vi "Test Upload to S3.vi"() -> ()   [LabVIEW 2019, in "SMO.Control Experiment.lvclass"]
uses:
  SMO.Control Experiment.lvclass
panel:
  out "Control Experiment out":refnum<class "SMO.Control Experiment.lvclass">
  in  "Control Experiment":refnum<class "SMO.Control Experiment.lvclass">
  in  "file to upload":path
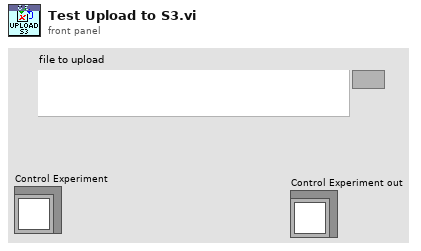
[diagram p1: front panel]
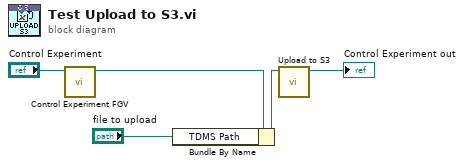
[diagram p0: block diagram]
diagram:
  n1 = call "Control Experiment FGV.vi"("Control Experiment"="Control Experiment") -> ("Control Experiment out"=w3:refnum<class "SMO.Control Experiment.lvclass">)  [unwired: 9 in, 1 out]
  n2 = Bundle By Name(cluster=w3, "TDMS Path"="file to upload") -> (w4:refnum<class "SMO.Control Experiment.lvclass">)
  n3 = call "Upload to S3.vi"("Control Experiment"=w4) -> ("Control Experiment out"=→"Control Experiment out":refnum<class "SMO.Control Experiment.lvclass">)  [unwired: 9 in, 1 out]
